vi "Tell Init Self.vi"(7 "Actor in":refnum<class "Actor.lvclass">, 10 "Input":T1) -> (0 "Error out":errorcluster, 1 "Told":bool, 5 "Actor out":refnum<class "Actor.lvclass">)   [LabVIEW 2020, in "_Template.lvlib" / "Templates.lvlib" / "TEMPLATE jettl Msg.lvlib"]
uses:
  TEMPLATE jettl Msg.lvlib
  jettl/jettl/jettl.lvlib
  jettl/jettl/Actor/Actor.lvclass
  Input.ctl
panel:
  # "This front panel should not be manipulated."
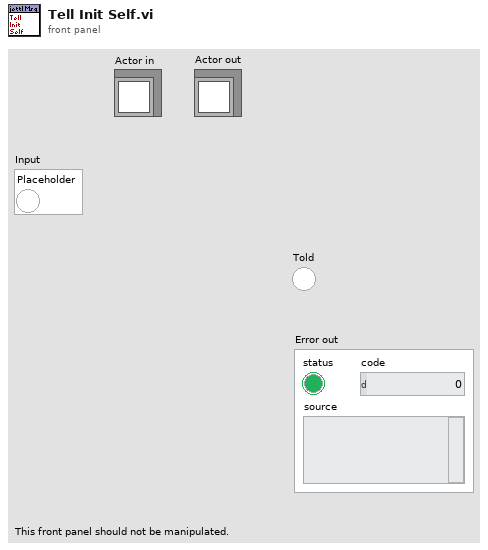
[diagram p1: front panel]
types:
  T1 = typedef "_Template.lvlib/Templates.lvlib/TEMPLATE jettl Msg.lvlib/Input.ctl" = cluster{"Placeholder":bool}
  T2 = typedef "jettl.lvlib/Msg.ctl" = cluster{"Msg":refnum<class "Msg.lvclass">, "Msg Input":refnum<class "Msg Input.lvclass">, "Msg Output":refnum<class "Msg Output.lvclass">, "Teller":T3}
  T3 = typedef "jettl.lvlib/Teller.ctl" = cluster{"Unified Actor Alias":string, "Unified Actor Relation":T4, "Absolute Time":timestamp, "Relative Time":dbl, "Msg DVR UID":i32}
  T4 = typedef "jettl.lvlib/Unified Actor Relation.ctl" = enum16{"Self", "Parent", "Child"}
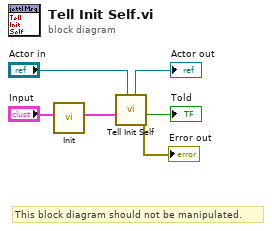
[diagram p0: block diagram]
diagram:
  # "This block diagram should not be manipulated."
  n1 = call "Init.vi"("Input"="Input") -> ("Msg"=w1:T2)  [unwired: 10 in]
  n2 = call "Tell Init Self.vi"("Actor in"="Actor in", "Msg"=w1) -> ("Error out"=→"Error out":errorcluster, "Told"=→"Told":bool, "Actor out"=→"Actor out":refnum<class "Actor.lvclass">)  [unwired: 7 in]
